vi "Test Untitled 2.vi"(8 "error in (no error)":errorcluster) -> (0 "error out":errorcluster, 3 "Pass?":bool)   [LabVIEW 2023]
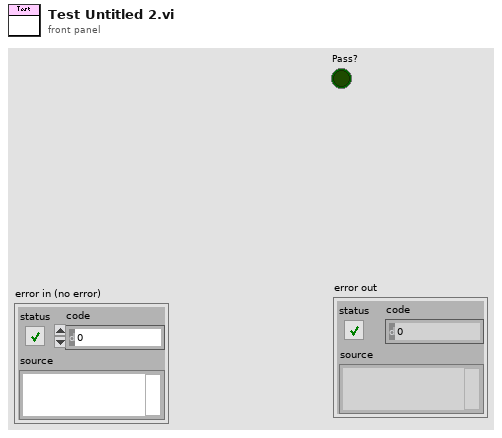
[diagram p1: front panel]
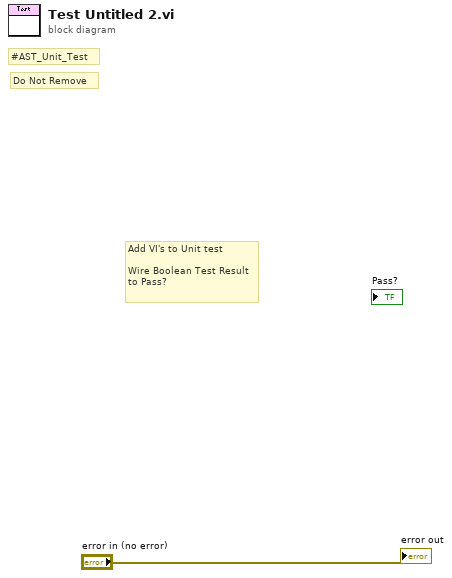
[diagram p0: block diagram]
diagram:
  # "Do Not Remove"
  # "#AST_Unit_Test"
  # "Add VI's to Unit test\n\nWire Boolean Test Result\nto Pass?"
  "error out" <- "error in (no error)"
